vi "tcp_服务器_发送.vi"(9 "远程端口或服务名称":u16=6314, 10 "原文件路径（使用对话框）":path=path "C:/Users/Administrator.2W964MZOGI5HE3B/Desktop/labview图片/105256rhad11pc5553vz5e.png", 11 "服务器网络地址":string="127.0.0.1") -> ()   [LabVIEW 2016, in "TCP文件传输系统.lvlib" / "TCP发送文件.lvlib"]
panel:
  out "当前步骤":T1(ring)
  out "error out":errorcluster
  out "错误输出":errorcluster
  out "已传百分比":string
  out "运行指示灯":bool=TRUE
  in  "分帧数(兆)":i64=2
  out "侦数":i32
  out "已发帧数":i32
  out "在发第几次":i32
  out "共发送次数":string
  in  "分一包（兆）":i64=40
  out "文件名称":string
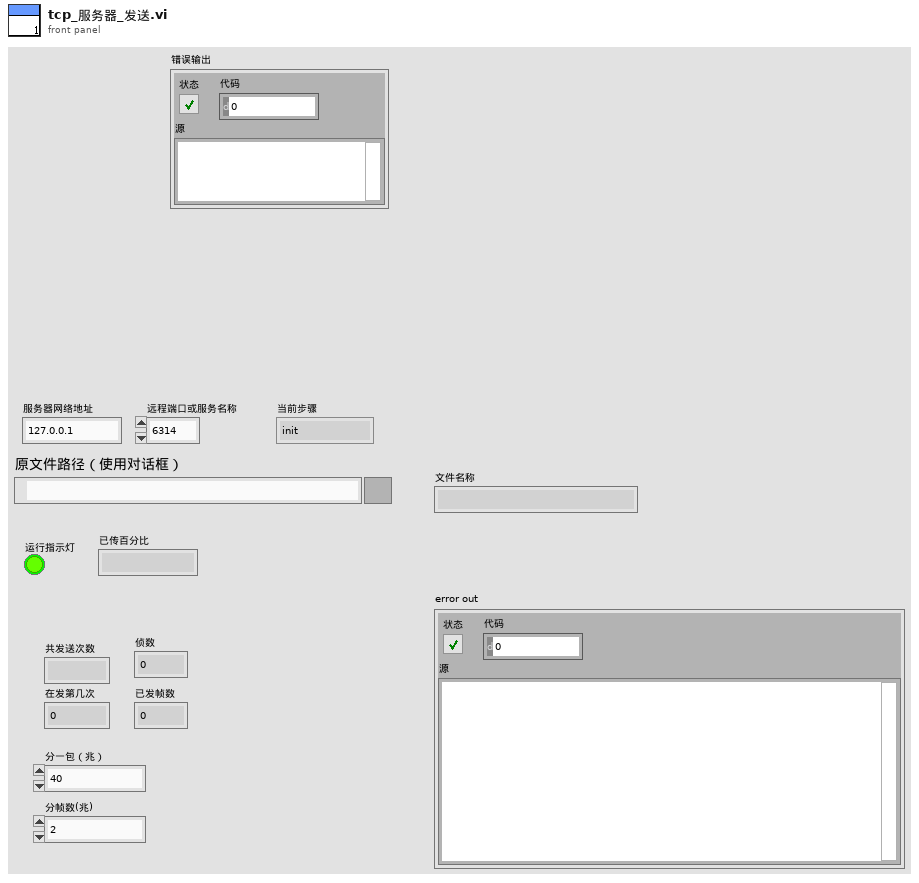
[diagram p1: front panel]
types:
  T1 = enum16{"init", "sendhead", "sendcontent", "sendsuccess", "over"}
  T2 = enum16{"open", "replace", "create", "open or create", "replace or create", "replace or create with confirmation"}
  T3 = cluster{"网络灯":bool, "发送中":bool, "已发送百分比":u8, "发送成功次数":dbl}
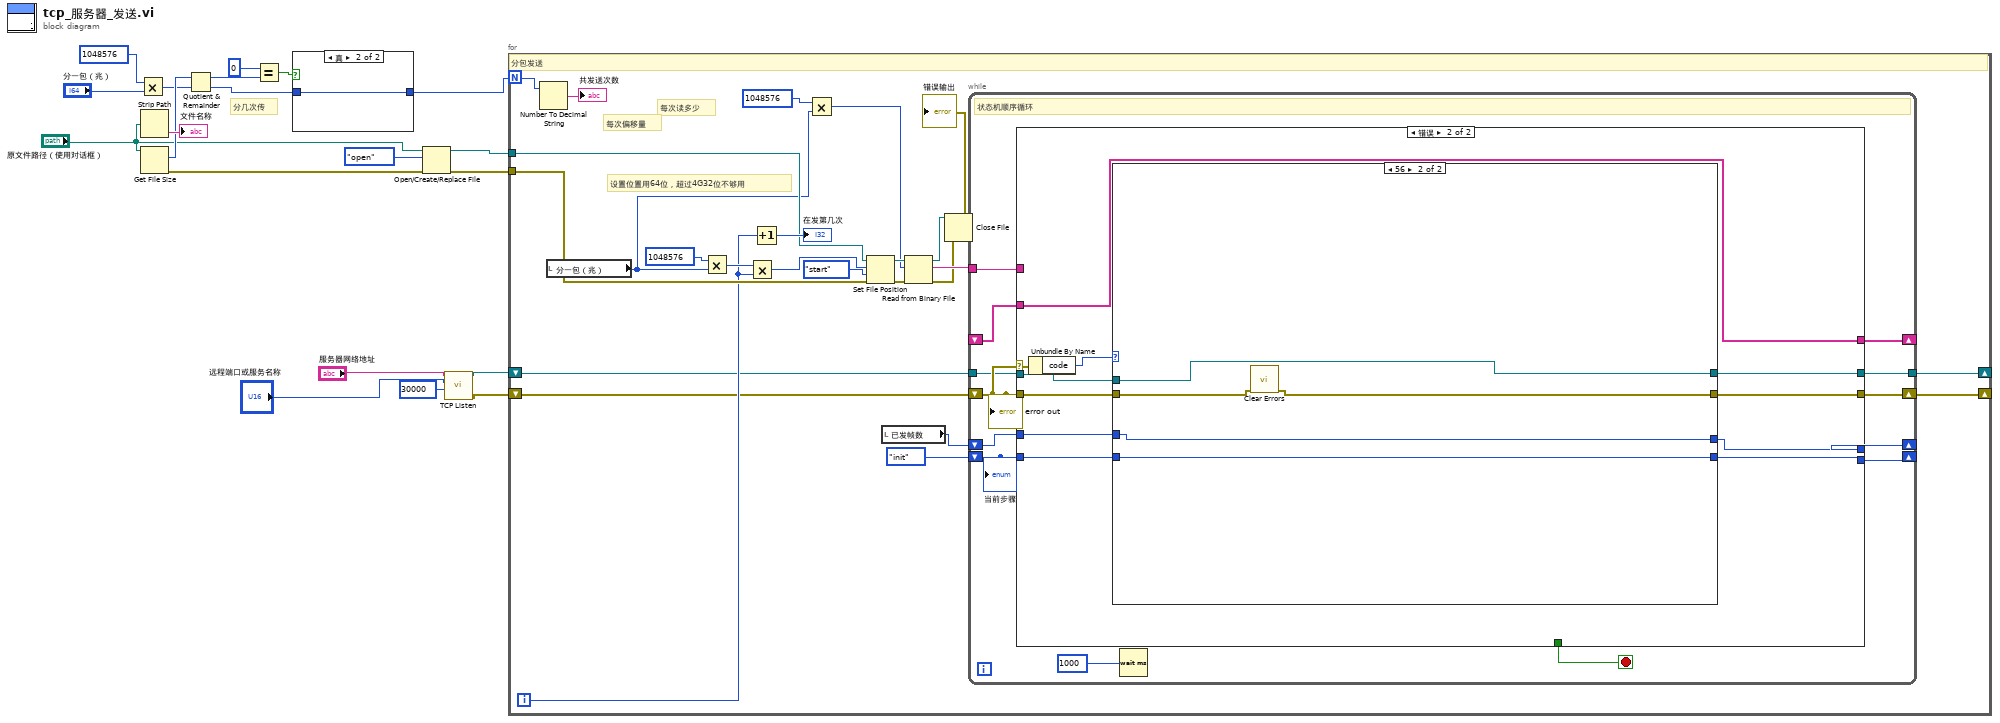
[diagram p0: block diagram]
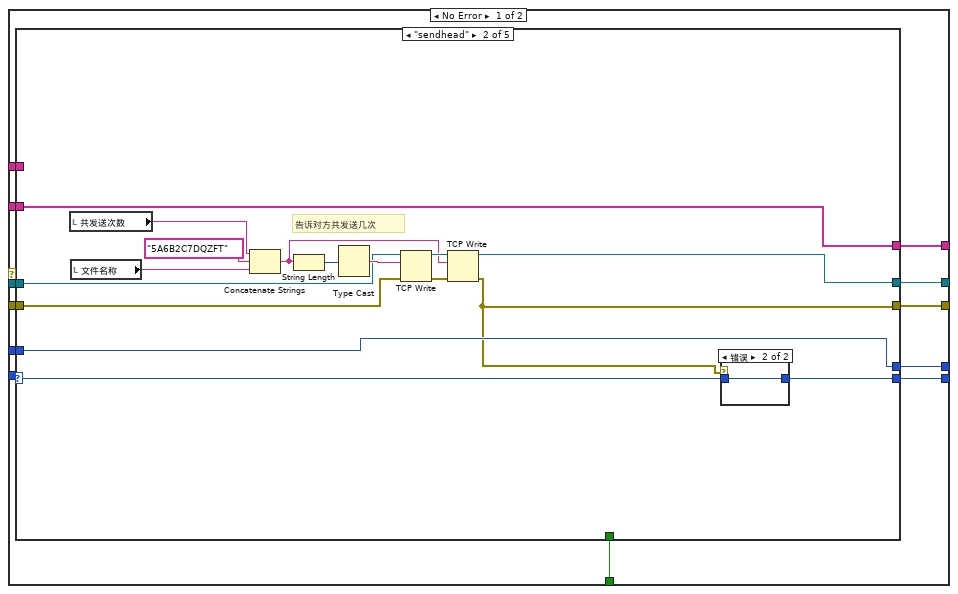
[diagram p2: hidden frame]
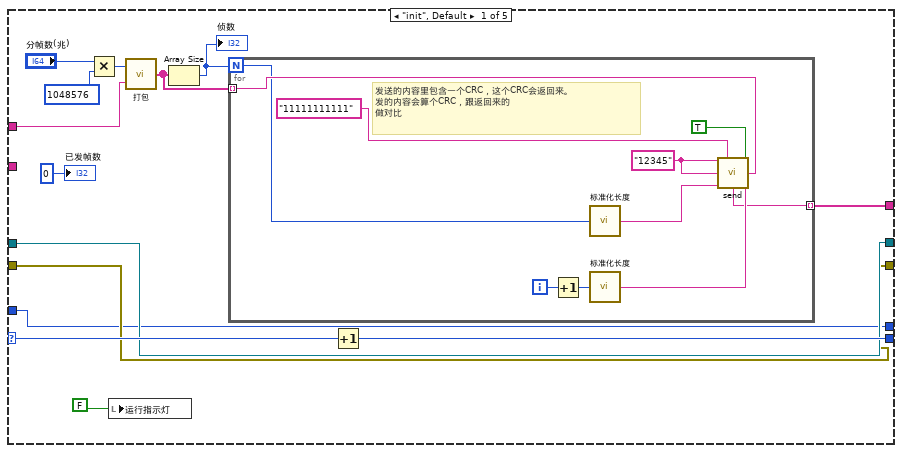
[diagram p3: hidden frame]
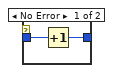
[diagram p4: hidden frame]
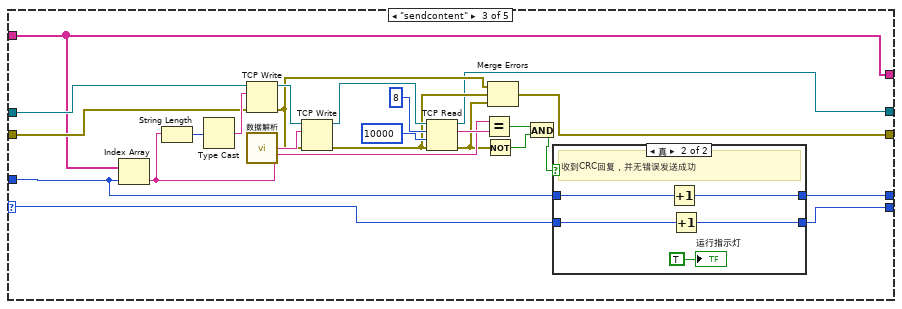
[diagram p5: hidden frame]
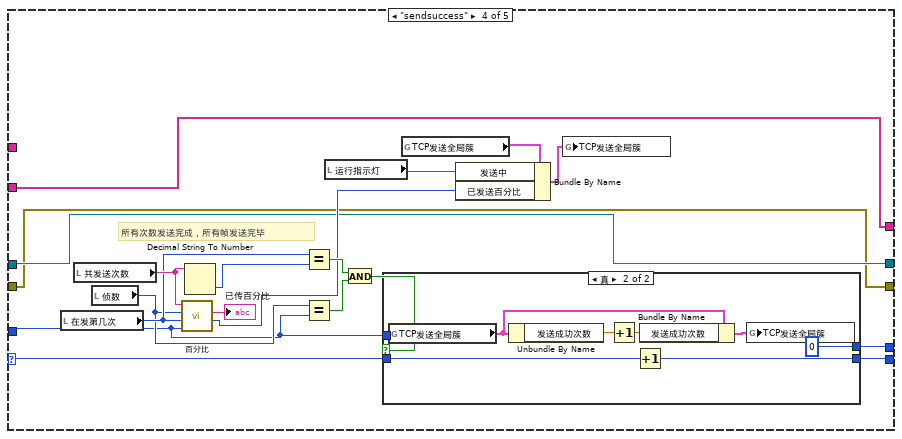
[diagram p7: hidden frame]
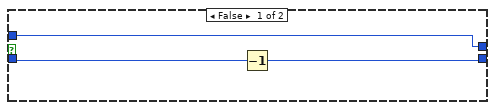
[diagram p8: hidden frame]
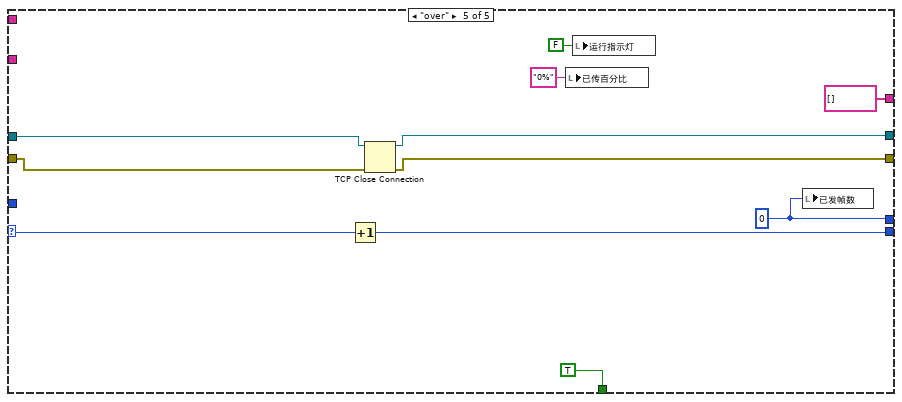
[diagram p9: hidden frame]
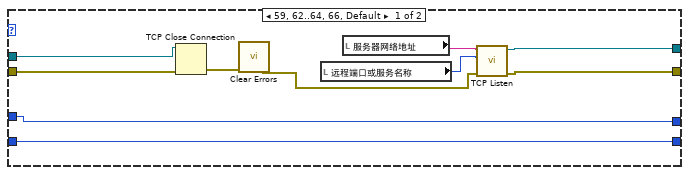
[diagram p10: hidden frame]
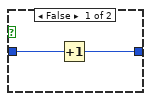
[diagram p11: hidden frame]
diagram:
  # "分几次传"
  n1 = Multiply(x=i64 1048576 ("y"), y="分一包（兆）") -> (x*y=w10:i64)
  n2 = Strip Path(path="原文件路径（使用对话框）") -> (name=→"文件名称":string)  [unwired: 1 out]
  n3 = Get File Size(file="原文件路径（使用对话框）") -> (size (in bytes)=w14:i64, 0:w15:errorcluster)  [unwired: 1 in, 1 out]
  n4 = Quotient & Remainder(x=w14, y=w10) -> (x-y*floor(x/y)=w19:i64, floor(x/y)=w16:i64)
  n5 = Equal?(x=0, y=w19) -> (x = y?=w17:bool)
  n6 = case shown="真" w17 {
    tunnel: [w21 w23] -> w8
    tunnel: w16 -> [w22 w23]
    frame False {
      n7 = Increment(x=w22) -> (x+1=w21:i64)
    }
    frame True {
    }
  }
  n8 = Open/Create/Replace File(file path (use dialog)="原文件路径（使用对话框）", error in=w15, operation (0:open)=T2."open" ("操作(0:open)")) -> (refnum out=w7:refnum<file>, error out=w6:errorcluster)  [unwired: 3 in, 1 out]
  n9 = call <vilib>:"TCP Listen.vi"("timeout ms (wait forever: -1)"=30000, "port"="远程端口或服务名称", "service name"="服务器网络地址") -> ("error out"=w3:errorcluster, "connection ID"=w4:refnum<k5>)  [unwired: 4 in, 3 out]
  n10 = for {
    N: w8 -> [w46]
    tunnel: w7 -> [w36]
    tunnel: w6 -> [w35]
    shift-right: [w29] -> _
    shift-left: w4 -> [w27]
    shift-right: [w28] -> _
    shift-left: w3 -> [w32]
    i -> [w34]
    # "设置位置用64位，超过4G32位不够用"
    # "每次读多少"
    # "每次偏移量"
    # "分包发送"
    n11 = Number To Decimal String(number=w46) -> (decimal integer string=→"共发送次数":string)  [unwired: 1 in]
    n12 = local read "分一包（兆）"() -> (w33:i64)
    n13 = Multiply(x=i64 1048576 ("偏移量（字节）（0）"), y=w33) -> (x*y=w39:i64)
    n14 = Multiply(x=w39, y=w34) -> (x*y=w42:i64)
    n15 = Increment(x=w34) -> (x+1=→"在发第几次":i32)
    n16 = Multiply(x=1048576 ("总数(1)"), y=w33) -> (x*y=w37:i64)
    n17 = Set File Position(offset (in bytes) (0)=w42, refnum=w36, from (0:start)=enum16{"start", "end", "current"}."start" ("自（0:起始）"), error in=w35) -> (refnum out=w44:refnum<file>, error out=w45:errorcluster)
    n18 = local read "已发帧数"() -> (w30:i32)
    n19 = Read from Binary File(8:w45, 10:w37, 11:w44) -> (0:w25:errorcluster, 2:w31:string, 3:w26:refnum<file>)  [unwired: 3 in, 1 out]
    n20 = Close File(refnum=w26, error in=w25) -> (error out=→"错误输出":errorcluster)  [unwired: 1 out]
    n21 = while {
      shift-right: [w60] -> _
      shift-left: T1."init" -> [w61]
      shift-right: [w54] -> w28
      shift-left: w32 -> [w56]
      tunnel: w31 -> [w57]
      shift-right: [w58] -> _
      shift-left: _ -> [w53]
      shift-right: [w51] -> _
      shift-left: w30 -> [w52]
      tunnel: w27 -> [w50]
      tunnel: [w55] -> w29
      stop <- w59 stop-if-true
      # "状态机顺序循环"
      n22 = case shown="错误" w56 {
        selector: w56 -> [_ w199]
        tunnel: w61 -> [w73 w193]
        tunnel: [w72 w192] -> w60
        tunnel: [w71 _] -> w59
        tunnel: [w70 w191] -> w58
        tunnel: w57 -> [w69 _]
        tunnel: w56 -> [w67 w197]
        tunnel: w50 -> [w68 w196]
        tunnel: [w64 w195] -> w55
        tunnel: [w65 w194] -> w54
        tunnel: w53 -> [w66 w191]
        tunnel: w52 -> [w63 w190]
        tunnel: [w62 w189] -> w51
        frame No Error {
          n23 = case shown="\"sendhead\"" w73 {
            selector: w73 -> [w87 w113 w119 w167 w188]
            tunnel: [w86 w112 w118 w166 w187] -> w72
            tunnel: [_ _ _ _ TRUE] -> w71
            tunnel: [w79 w101 w117 w149 string[] []] -> w70
            tunnel: w69 -> [w78 _ _ _ _]
            tunnel: w68 -> [w77 w103 w125 w151 w184]
            tunnel: w67 -> [w76 w102 w126 w150 w183]
            tunnel: w66 -> [_ w101 w117 w149 _]
            tunnel: [w76 w98 w123 w150 w181] -> w65
            tunnel: [w77 w100 w124 w151 w182] -> w64
            tunnel: w63 -> [w75 w99 w121 w152 _]
            tunnel: [w75 w99 w120 w153 w185] -> w62
            frame "init", Default {
              n24 = Multiply(x="分帧数(兆)", y=i64 1048576) -> (x*y=w83:i64)
              n25 = local write "运行指示灯"(FALSE ("运行指示灯")) -> ()
              n26 = call "打包.vi"("总内容"=w78, "分包大小"=w83) -> ("分包数组"=w82:string[])
              n27 = Array Size(array=w82) -> (size(s)=w84:i32)
              "侦数" <- w84
              n28 = for {
                N: w84 -> [w92]
                tunnel: w82 -> [w97] mode=indexing
                tunnel: [w90] -> w79 mode=indexing
                i -> [w96]
                w89 = "12345" ("内容说明（文件名）")
                # "发送的内容里包含一个CRC，这个CRC会返回来。\n发的内容会算个CRC，跟返回来的\n做对比"
                n29 = Increment(x=w96) -> (x+1=w91:i32)
                n30 = call "标准化长度.vi"("原长度"=w92) -> ("标准化长度"=w95:string)
                n31 = call "标准化长度.vi"("原长度"=w91) -> ("标准化长度"=w94:string)
                n32 = call "send.vi"("内容标识"=w89, "时标"="11111111111", "发送"=TRUE, "内容说明（文件名）"=w89, "帧内容"=w97, "帧数"=w95, "帧号"=w94) -> ("连接的字符串"=w90:string)  [unwired: 6 in, 2 out]
              }
              n33 = Increment(x=w87) -> (x+1=w86:T1)
              "已发帧数" <- 0 ("数值")
            }
            frame "sendhead" {
              # "告诉对方共发送几次"
              n34 = local read "共发送次数"() -> (w108:string)
              n35 = local read "文件名称"() -> (w109:string)
              n36 = Concatenate Strings(w108, "5A6B2C7DQZFT" ("字符串"), w109) -> (w104:string)
              n37 = String Length(string=w104) -> (length=w111:i32)
              n38 = Type Cast(x=w111) -> (*(type *) &x=w105:string)  [unwired: 1 out]
              n39 = TCP Write(connection ID=w103, data in=w105, error in (no error)=w102) -> (connection ID out=w106:refnum<k5>, error out=w107:errorcluster)  [unwired: 2 out]
              n40 = TCP Write(connection ID=w106, data in=w104, error in (no error)=w107) -> (connection ID out=w100:refnum<k5>, error out=w98:errorcluster)  [unwired: 2 out]
              n41 = case shown="错误" w98 {
                tunnel: w113 -> [w115 w116]
                tunnel: [w114 w116] -> w112
                frame No Error {
                  n42 = Increment(x=w115) -> (x+1=w114:T1)
                }
                frame Error {
                }
              }
            }
            frame "sendcontent" {
              n43 = Index Array(array=w117, index=w121) -> (element=w136:string)
              n44 = String Length(string=w136) -> (length=w140:i32)
              n45 = Type Cast(x=w140) -> (*(type *) &x=w137:string)  [unwired: 1 out]
              n46 = TCP Write(connection ID=w125, data in=w137, error in (no error)=w126) -> (connection ID out=w141:refnum<k5>, error out=w128:errorcluster)  [unwired: 2 out]
              n47 = call "数据解析.vi"("data in"=w136) -> ("data out"=w135:string, "CRC"=w133:string)  [unwired: 4 in, 9 out]
              n48 = TCP Write(connection ID=w141, data in=w135, error in (no error)=w128) -> (connection ID out=w139:refnum<k5>, error out=w127:errorcluster)  [unwired: 2 out]
              n49 = TCP Read(connection ID=w139, bytes to read=8 ("读取的字节"), error in (no error)=w127, 9:10000 ("超时毫秒(25000)")) -> (connection ID out=w124:refnum<k5>, data out=w134:string, error out=w129:errorcluster)  [unwired: 1 in]
              n50 = Equal?(x=w133, y=w134) -> (x = y?=w131:bool)
              n51 = Not(x=w129) -> (.not. x?=w130:bool)
              n52 = Merge Errors(w128, w127, w129) -> (w123:errorcluster)
              n53 = And(x=w131, y=w130) -> (x .and. y?=w122:bool)
              n54 = case shown="真" w122 {
                tunnel: w121 -> [w143 w147]
                tunnel: [w143 w146] -> w120
                tunnel: w119 -> [w142 w145]
                tunnel: [w142 w144] -> w118
                frame False {
                  # "未收到正确回复，或超时"
                }
                frame True {
                  # "收到CRC回复，并无错误发送成功"
                  n55 = Increment(x=w147) -> (x+1=w146:i32)
                  n56 = Increment(x=w145) -> (x+1=w144:T1)
                  "运行指示灯" <- TRUE
                }
              }
            }
            frame "sendsuccess" {
              # "所有次数发送完成，所有帧发送完毕"
              n57 = local read "在发第几次"() -> (w163:i32)
              n58 = local read "共发送次数"() -> (w164:string)
              n59 = local read "侦数"() -> (w161:i32)
              n60 = call "百分比.vi"("已发帧数 2"=w152, "发第几次"=w163, "帧数"=w161, "共发送次数"=w164) -> ("已发送百分比"=w154:u8, "已传百分比"=→"已传百分比":string)  [unwired: 6 in]
              n61 = Decimal String To Number(string=w164) -> (number=w162:i32)  [unwired: 2 in, 1 out]
              n62 = Equal?(x=w163, y=w162) -> (x = y?=w160:bool)
              n63 = Equal?(x=w161, y=w152) -> (x = y?=w159:bool)
              n64 = local read "运行指示灯"() -> (w155:bool)
              n65 = And(x=w160, y=w159) -> (x .and. y?=w158:bool)
              n66 = case shown="真" w158 {
                tunnel: w167 -> [w170 w177]
                tunnel: [w169 w176] -> w166
                tunnel: [w168 0 ("已发帧数")] -> w153
                tunnel: w152 -> [w168 _]
                frame False {
                  n67 = Decrement(x=w170) -> (x-1=w169:T1)
                }
                frame True {
                  n68 = global read "全局变量1.vi" "TCP发送全局簇"() -> (w172:T3)
                  n69 = Unbundle By Name(w172) -> ("发送成功次数"=w173:dbl)
                  n70 = Increment(x=w173) -> (x+1=w174:dbl)
                  n71 = Increment(x=w177) -> (x+1=w176:T1)
                  n72 = Bundle By Name(cluster=w172, "发送成功次数"=w174) -> (w175:T3)
                  n73 = global write "全局变量1.vi" "TCP发送全局簇"(w175) -> ()
                }
              }
              n74 = global read "全局变量1.vi" "TCP发送全局簇"() -> (w156:T3)
              n75 = Bundle By Name(cluster=w156, "发送中"=w155, "已发送百分比"=w154) -> (w157:T3)
              n76 = global write "全局变量1.vi" "TCP发送全局簇"(w157) -> ()
            }
            frame "over" {
              w185 = 0
              n77 = Increment(x=w188) -> (x+1=w187:T1)
              n78 = TCP Close Connection(connection ID=w184, error in (no error)=w183) -> (connection ID out=w182:refnum<k5>, error out=w181:errorcluster)  [unwired: 1 in]
              n79 = local write "已传百分比"("0%" ("已传百分比")) -> ()
              n80 = local write "运行指示灯"(FALSE ("运行指示灯")) -> ()
              n81 = local write "已发帧数"(w185) -> ()
            }
          }
        }
        frame Error {
          n82 = Unbundle By Name(w199) -> ("code"=w198:i32)
          n83 = case shown="56" w198 {
            tunnel: w197 -> [w209 w212]
            tunnel: w196 -> [w208 w211]
            tunnel: [w201 w211] -> w195
            tunnel: [w202 w210] -> w194
            tunnel: w193 -> [w200 w214]
            tunnel: [w200 w214] -> w192
            tunnel: w190 -> [w206 w213]
            tunnel: [w206 w213] -> w189
            frame 59, 62..64, 66, Default {
              n84 = TCP Close Connection(connection ID=w208, error in (no error)=w209) -> (error out=w207:errorcluster)  [unwired: 1 in, 1 out]
              n85 = call <vilib>:"Clear Errors.vi"("error in (no error)"=w207) -> ("error out"=w203:errorcluster)  [unwired: 5 in, 1 out]
              n86 = local read "远程端口或服务名称"() -> (w204:u16)
              n87 = local read "服务器网络地址"() -> (w205:string)
              n88 = call <vilib>:"TCP Listen.vi"("error in (no error)"=w203, "port"=w204, "service name"=w205) -> ("error out"=w202:errorcluster, "connection ID"=w201:refnum<k5>)  [unwired: 4 in, 3 out]
            }
            frame 56 {
              n89 = call <vilib>:"Clear Errors.vi"("error in (no error)"=w212) -> ("error out"=w210:errorcluster)  [unwired: 5 in, 1 out]
            }
          }
        }
      }
      n90 = Wait (ms)(milliseconds to wait=u32 1000 ("等待时间（毫秒）")) -> ()  [unwired: 1 out]
      "error out" <- w56
      "当前步骤" <- w61
    }
  }
